vi "Freq2Time.vi"(8 "error in (no error)":errorcluster, 10 "Int. Time Unit":enum16{"sec", "us", "ms"}(ring), 11 "Sample rate (Hz)":dbl=5000.0 min=0.0 step=100.0 format="%.2p") -> (0 "error out":errorcluster, 2 "Int.  time [unit]":dbl=5000.0 step=100.0, 3 "New Sample rate (Hz)":dbl=5000.0 min=0.0 step=100.0 format="%.2p")   [LabVIEW 2018, in "Timing.lvlib"]
doc: "Converts the input frequency (Hz) into an integeral value of seleted time unit and corresponding frequency."
uses:
  Timing.lvlib
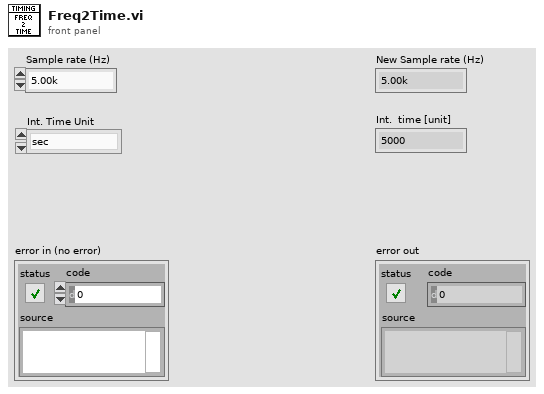
[diagram p1: front panel]
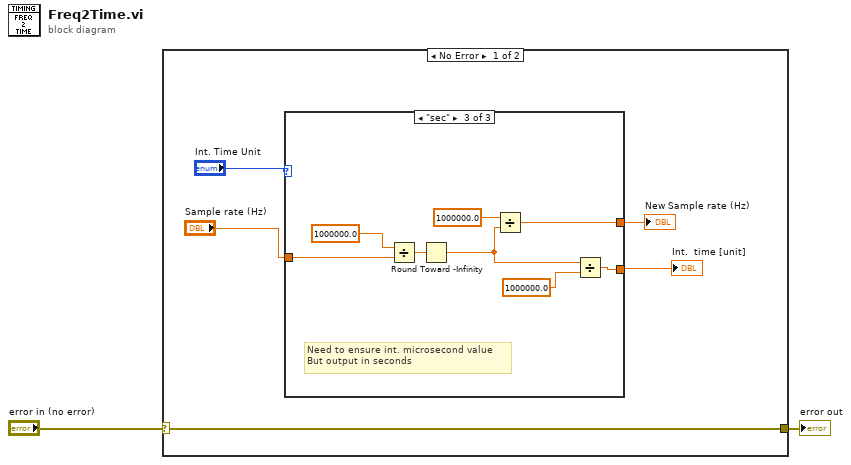
[diagram p0: block diagram]
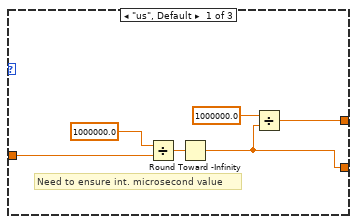
[diagram p2: hidden frame]
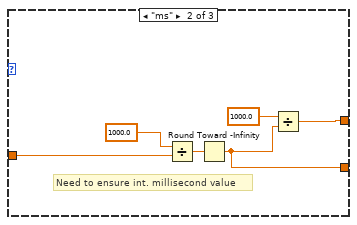
[diagram p3: hidden frame]
diagram:
  n1 = case shown="No Error" "error in (no error)" {
    selector: "error in (no error)" -> [w6 w28]
    tunnel: [w6 w28] -> w1
    frame No Error {
      n2 = case shown="\"sec\"" "Int. Time Unit" {
        tunnel: "Sample rate (Hz)" -> [w13 w16 w24]
        tunnel: [w9 w15 w23] -> w4
        tunnel: [w8 w14 w22] -> w3
        frame "us", Default {
          # "Need to ensure int. microsecond value"
          n3 = Divide(x=1000000.0, y=w13) -> (x/y=w11:dbl)
          n4 = Round Toward -Infinity(1:w11) -> (0:w8:dbl)
          n5 = Divide(x=1000000.0, y=w8) -> (x/y=w9:dbl)
        }
        frame "ms" {
          # "Need to ensure int. millisecond value"
          n6 = Divide(x=1000.0, y=w16) -> (x/y=w18:dbl)
          n7 = Round Toward -Infinity(1:w18) -> (0:w14:dbl)
          n8 = Divide(x=1000.0, y=w14) -> (x/y=w15:dbl)
        }
        frame "sec" {
          # "Need to ensure int. microsecond value\nBut output in seconds"
          n9 = Divide(x=1000000.0, y=w24) -> (x/y=w26:dbl)
          n10 = Round Toward -Infinity(1:w26) -> (0:w21:dbl)
          n11 = Divide(x=1000000.0, y=w21) -> (x/y=w23:dbl)
          n12 = Divide(x=w21, y=1000000.0) -> (x/y=w22:dbl)
        }
      }
      "New Sample rate (Hz)" <- w4
      "Int.  time [unit]" <- w3
    }
    frame Error {
    }
  }
  "error out" <- w1
